vi "Replace Array Elements - variant.vi"(4 "new elements (none)":variant[](array[variant]), 5 "indices (none)":i32[](array[numeric])=[3, 5], 7 "1D Array":variant[](array[variant])) -> (2 "output array":variant[](array[variant]))   [LabVIEW 2020]
doc: "Replaces elements in a 1-dim array at the specified indices. This is a list-based version of the built-in \"Replace Array Subset\"."
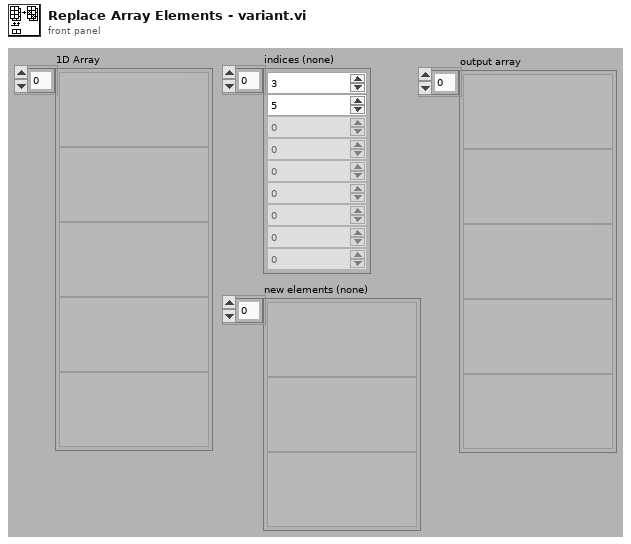
[diagram p1: front panel]
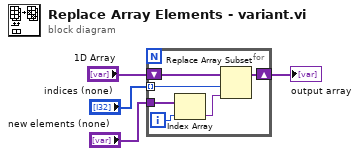
[diagram p0: block diagram]
diagram:
  n1 = for {
    tunnel: "new elements (none)" -> [w8]
    shift-right: [w9] -> w3
    shift-left: "1D Array" -> [w10]
    tunnel: "indices (none)" -> [w6] mode=indexing
    i -> [w5]
    n2 = Index Array(array=w8, index=w5) -> (element=w7:variant)
    n3 = Replace Array Subset(array=w10, new element=w7, index=w6) -> (w9:variant[])
  }
  "output array" <- w3
